vi "joystick1.vi"() -> ()   [LabVIEW 2016]
uses:
  <vilib>/Utility/inputDevices.llb/joystickAcquire.vi
  <vilib>/Utility/inputDevices.llb/closeJoystick.vi
panel:
  in  "Stop Button":bool
  out "direction info":T1
  out "button info":T2
  out "axis info":T3
  out "mouse info":T4(array[cluster])
  out "joystick info":T5(array[cluster])
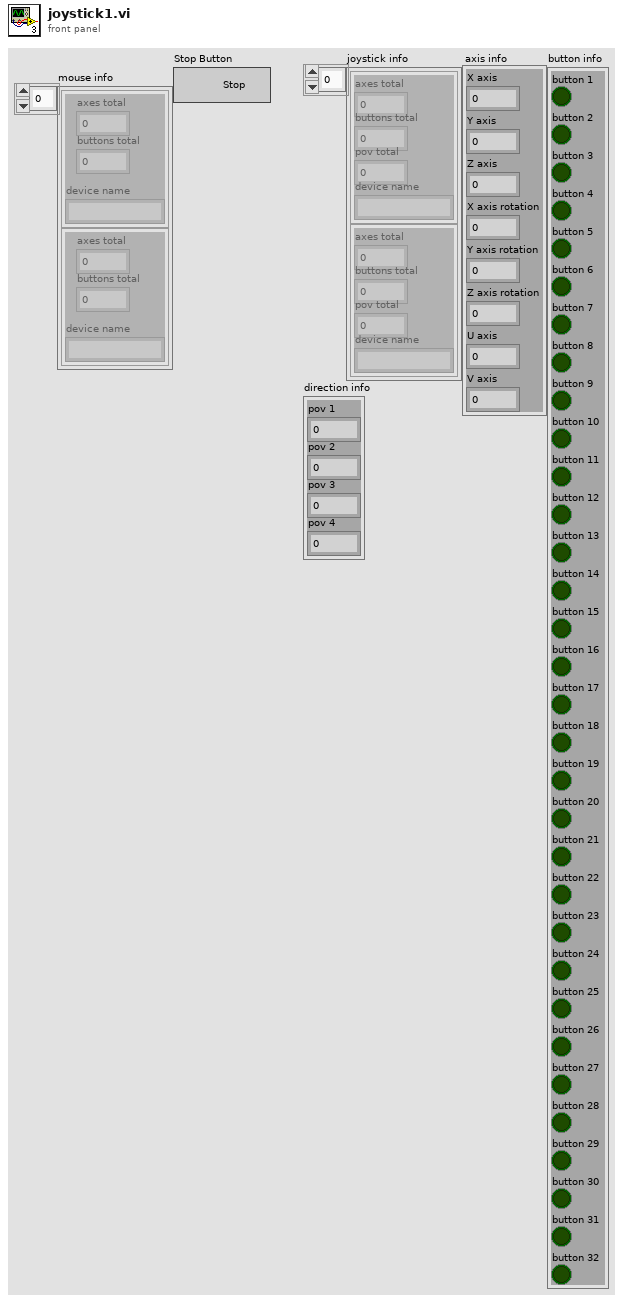
[diagram p1: front panel]
types:
  T1 = cluster{"pov 1":i32, "pov 2":i32, "pov 3":i32, "pov 4":i32}
  T2 = cluster{"button 1":bool, "button 2":bool, "button 3":bool, "button 4":bool, "button 5":bool, "button 6":bool, "button 7":bool, "button 8":bool, "button 9":bool, "button 10":bool, "button 11":bool, "button 12":bool, "button 13":bool, "button 14":bool, "button 15":bool, "button 16":bool, "button 17":bool, "button 18":bool, "button 19":bool, "button 20":bool, "button 21":bool, "button 22":bool, "button 23":bool, "button 24":bool, "button 25":bool, "button 26":bool, "button 27":bool, "button 28":bool, "button 29":bool, "button 30":bool, "button 31":bool, "button 32":bool}
  T3 = cluster{"X axis":i32, "Y axis":i32, "Z axis":i32, "X axis rotation":i32, "Y axis rotation":i32, "Z axis rotation":i32, "U axis":i32, "V axis":i32}
  T4 = cluster{"axes total":u32, "buttons total":u32, "device name":string}[]
  T5 = cluster{"axes total":u32, "buttons total":u32, "pov total":u32, "device name":string}[]
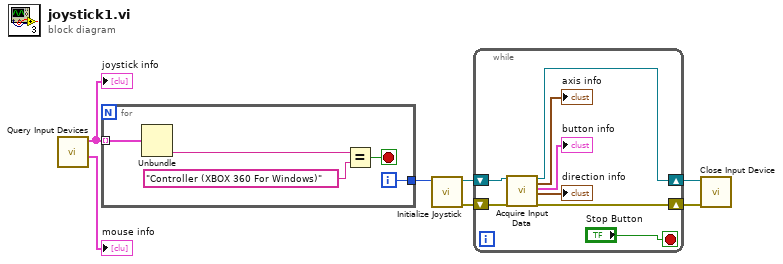
[diagram p0: block diagram]
diagram:
  n1 = call <vilib>:"Query Input Devices.vi"() -> ("mouse info"=→"mouse info":T4, "joystick info"=w6:T5)  [unwired: 8 in, 2 out]
  "joystick info" <- w6
  n2 = for {
    tunnel: w6 -> [w12] mode=indexing
    tunnel: [w8] -> w5
    i -> [w8]
    stop <- w9 stop-if-true
    n3 = Unbundle(w12) -> ("device name"=w10:string)  [unwired: 3 out]
    n4 = Equal?(x=w10, y="Controller (XBOX 360 For Windows)") -> (x = y?=w9:bool)
  }
  n5 = call <vilib>:"Initialize Joystick.vi"("device index"=w5) -> ("error out"=w3:errorcluster, "device ID"=w4:refnum<k1>)  [unwired: 9 in]
  n6 = while {
    shift-right: [w17] -> w1
    shift-left: w4 -> [w20]
    shift-right: [w18] -> w2
    shift-left: w3 -> [w19]
    stop <- "Stop Button" stop-if-true
    n7 = call-poly <vilib>:"Acquire Input Data.vi"("device ID"=w20, "error in (no error)"=w19) -> ("device ID"=w17:refnum<k1>, "axis info"=→"axis info":T3, "button info"=→"button info":T2, "direction info"=→"direction info":T1, "error out"=w18:errorcluster)  [unwired: 13 in]
  }
  n8 = call-poly <vilib>:"Close Input Device.vi"("error in (no error)"=w2, "device ID"=w1) -> ()  [unwired: 8 in, 1 out]
